vi "LIDAR Data Loop.vi"() -> ()   [LabVIEW 2011]
uses:
  <vilib>/Platform/TimedLoop/XDataNode/timing_clust.ctl
  <vilib>/Platform/TimedLoop/XDataNode/nitl_modes.ctl
  <vilib>/Platform/TimedLoop/XDataNode/wakeup.ctl
  <instrlib>/Hokuyo URG Series/Public/Initialize-Standard.vi
  <vilib>/Platform/TimedLoop/XDataNode/XDataNode.xnode
  <vilib>/Platform/TimedLoop/XDataNode/XDNodeRunTimeDep.lvlib
  <instrlib>/Hokuyo URG Series/Hokuyo URG Series.lvlib
panel:
  in  "error in":errorcluster
  in  "VISA resource name":refnum<visa-resource-name>
  in  "Debug":bool
  out "LIDAR Data":cluster{"Magnitude":dbl[], "Direction":dbl[]}
  in  "end point (135°)":dbl=135.0
  in  "start point (-135°)":dbl=-135.0
  out "error out":errorcluster
  in  "protocol":u32(ring)=2 items=["Convert to Latest", "SCIP 1.1", "SCIP 2.0"]
  in  "stop?":bool
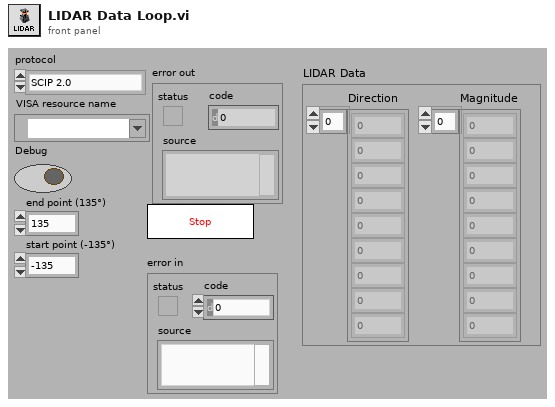
[diagram p1: front panel]
types:
  T1 = typedef "XDNodeRunTimeDep.lvlib/timing_clust.ctl" = cluster{"Expected End [f-1]":u64, "Actual End [f-1]":u64, "Finished Late? [f-1]":bool, "Expected End [i-1]":u64, "Actual End [i-1]":u64, "Finished Late? [i-1]":bool, "Expected Start [i]":u64, "Actual Start [i]":u64, "Expected Start [f]":u64, "Actual Start [f]":u64, "Source Name":string, "Structure Name":string, "Period":i64, "Deadline":i64, "Offset":i64, "Start":i64, "Priority":i32, "Timeout":i32, "Mode":T2, "Wakeup Reason":T3, "Error":errorcluster, "Source Type":string, "Secondary Source Type":string, "Global End Time":u64, "Global Start Time":u64, "Frame Duration":u64, "Iteration Duration":u64, "Assigned CPU":i32, "I/O Scan Engine Mode":u32}
  T2 = typedef "XDNodeRunTimeDep.lvlib/nitl_modes.ctl" = enum32{"No Change", "Process missed periods, maintain original phase", "Discard missed periods, maintain original phase", "Process missed periods, ignore original phase", "Discard missed periods, ignore original phase"}
  T3 = typedef "XDNodeRunTimeDep.lvlib/wakeup.ctl" = enum32{"Normal", "Aborted", "Asynchronous wakeup", "Timing source error", "Timed loop error", "Timeout"}
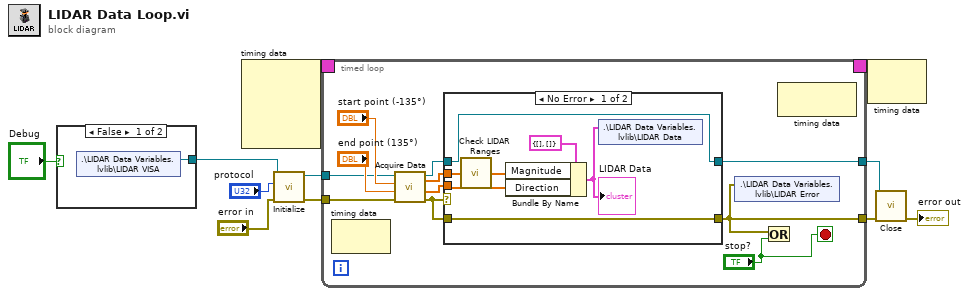
[diagram p0: block diagram]
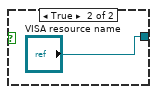
[diagram p2: hidden frame]
diagram:
  n1 = case shown="False" "Debug" {
    tunnel: [w12 "VISA resource name"] -> w5
    frame False {
      n2 = shared-variable ".\\LIDAR Data Variables.lvlib\\LIDAR VISA"() -> (w12:refnum<visa-resource-name>)  [unwired: 1 in, 1 out]
    }
    frame True {
    }
  }
  n3 = node-c288() -> (w11:T1)  [unwired: 4 out]
  n4 = call-poly <instrlib>:"Initialize.vi"("error in (no error)"="error in", "Protocol (2: SCIP 2.0)"="protocol", "VISA resource name"=w5) -> ("error out"=w3:errorcluster, "VISA resource name out"=w4:refnum<visa-resource-name>)  [unwired: 7 in]
  n5 = timed-loop {
    timing: w11 -> [_]
    timing-out: [_] -> w10
    tunnel: w4 -> [w20]
    tunnel: [w18] -> w8
    tunnel: [w15] -> w7
    tunnel: w3 -> [w16]
    stop <- "stop?" stop-if-true
    n6 = node-c288() -> ()  [unwired: 2 out]
    n7 = call <instrlib>:"Acquire Data.vi"("error in (no error)"=w16, "End Point (120°)"="end point (135°)", "Start Point (-120°)"="start point (-135°)", "VISA resource name"=w20) -> ("error out"=w17:errorcluster, "Direction"=w23:dbl[], "Magnitude"=w24:dbl[], "VISA resource name out"=w19:refnum<visa-resource-name>)  [unwired: 4 in]
    n8 = case shown="No Error" w17 {
      selector: w17 -> [_ w32]
      tunnel: w24 -> [w25 _]
      tunnel: w23 -> [w28 _]
      tunnel: w19 -> [w31 w33]
      tunnel: [w31 w33] -> w18
      tunnel: [w30 w32] -> w15
      tunnel: w17 -> [w30 _]
      frame No Error {
        n9 = call "Check LIDAR Ranges.vi"("Magnitude"=w25) -> ("Magnitude out"=w26:dbl[])  [unwired: 4 in]
        n10 = Bundle By Name(cluster=cluster{"Magnitude":dbl[], "Direction":dbl[]} {"Magnitude"=[], "Direction"=[]} ("LIDAR Data"), "Magnitude"=w26, "Direction"=w28) -> (w27:cluster{"Magnitude":dbl[], "Direction":dbl[]})
        "LIDAR Data" <- w27
        n11 = shared-variable ".\\LIDAR Data Variables.lvlib\\LIDAR Data"(w27) -> ()  [unwired: 1 in, 1 out]
      }
      frame Error {
      }
    }
    n12 = shared-variable ".\\LIDAR Data Variables.lvlib\\LIDAR Error"(w15) -> ()  [unwired: 1 in, 1 out]
    n13 = Or(x=w15, y="stop?") -> ()  [unwired: 1 out]
    n14 = node-c288() -> ()  [unwired: 2 out]
  }
  n15 = node-c288(w10) -> ()  [unwired: 1 out]
  n16 = call <instrlib>:"Close.vi"("error in (no error)"=w7, "VISA resource name"=w8) -> ("error out"=→"error out":errorcluster)  [unwired: 9 in]
